vi "Get TX Message.vi"(8 "error in (no error)":errorcluster, 11 "RxTx in":refnum<class "RxTx.lvclass">) -> (0 "error out":errorcluster, 3 "RxTx out":refnum<class "RxTx.lvclass">)   [LabVIEW 2018, in "RxTx.lvclass"]
uses:
  RxTx.lvclass
  RxTx.lvclass/RxTx.ctl
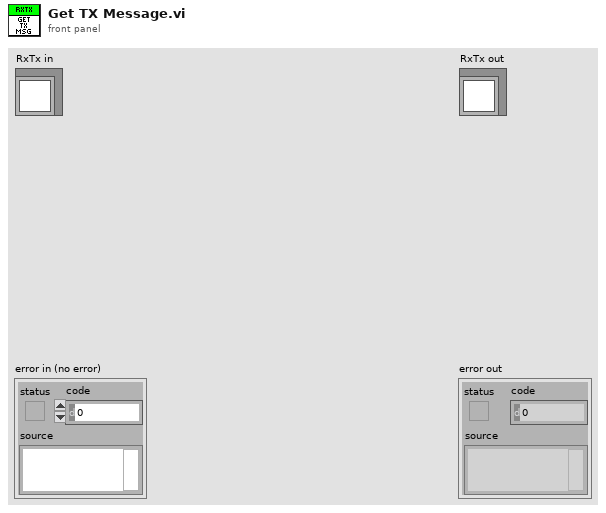
[diagram p1: front panel]
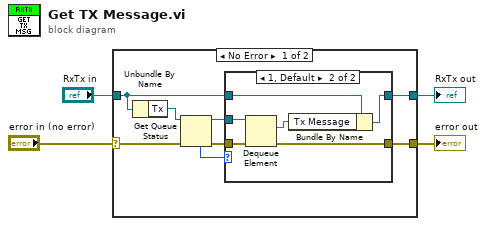
[diagram p0: block diagram]
diagram:
  n1 = case shown="No Error" "error in (no error)" {
    selector: "error in (no error)" -> [w8 w22]
    tunnel: [w6 w22] -> w2
    tunnel: [w11 w21] -> w1
    tunnel: "RxTx in" -> [w12 w21]
    frame No Error {
      n2 = Unbundle By Name(w12) -> ("Tx"=w9:refnum<queue>)
      n3 = Get Queue Status(queue=w9, error in (no error)=w8) -> (queue out=w5:refnum<queue>, error out=w7:errorcluster, # elements in queue=w10:i32)  [unwired: 1 in, 5 out]
      n4 = case shown="1, Default" w10 {
        tunnel: w12 -> [w13 w20]
        tunnel: [w13 w19] -> w11
        tunnel: w7 -> [w14 w17]
        tunnel: [w14 w16] -> w6
        tunnel: w5 -> [_ w15]
        frame 0 {
        }
        frame 1, Default {
          n5 = Dequeue Element(queue=w15, error in (no error)=w17) -> (element=w18:string, error out=w16:errorcluster)  [unwired: 1 in, 2 out]
          n6 = Bundle By Name(cluster=w20, "Tx Message"=w18) -> (w19:refnum<class "RxTx.lvclass">)
        }
      }
    }
    frame Error {
    }
  }
  "error out" <- w2
  "RxTx out" <- w1
